vi "Write_Results_file.vi"(0 "Experiment start time":dbl, 1 "Experiment End time":dbl, 3 "Setup filename":string) -> ()   [LabVIEW 2022 SP3]
uses:
  Controls/Post_Process.ctl
  Controls/Inst_type.ctl
  Controls/Global_mode.ctl
  <vilib>/Analysis/baseanly.llb/Mean (DBL).vi
  Globals/Meas_global.vi
  Globals/Trav_pos_global.vi
  Globals/Dynamic_call_global.ph.vi
  <vilib>/Analysis/NI_AALBase.lvlib
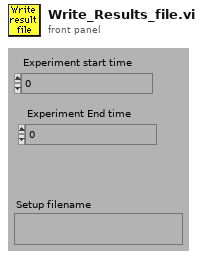
[diagram p1: front panel]
types:
  T1 = typedef "Post_Process.ctl" = enum16{"Take New Data", "Post Process Raw Data File"}
  T2 = enum16{"Save no data", "Save data in new files", "Save data in existing files"}
  T3 = typedef "Inst_type.ctl" = enum16{"Raw voltage", "Raw with zero offsetting", "Propeller anemometer", "Pressure Transducer", "Pitot-static tube", "Hot wire", "Cross wire 1", "Cross wire 2", "Generic Linear", "Generic Polynomial", "Generic BackPoly", "Fast FID", "Thermocouple", "Cold wire", "Pulsed Wire", "LDA Vel", "LDA Tran time", "LDA Arr time", "Microphone"}
  T4 = typedef "Global_mode.ctl" = enum16{"Read Global", "Load Global From File", "Write Global to File"}
  T5 = typedef "Analysis_info_cluster.ctl" = cluster{"Colour":u32, "Inst type":T3, "Inst name":string, "Symbol":string, "Code name":string, "Extra Info":string, "Inst Array":T6, "Extra Titles":string[], "Extra Values":string[], "U":dbl, "u^2":dbl, "u^3":dbl, "u^4":dbl, "Skew_u":dbl, "Kurt_u":dbl, "Sd Error in Mean":dbl, "% u'/U":dbl, "X":dbl, "Y":dbl, "Z":dbl, "Timescale integral Estimate":dbl, "Sd Error in Variance":dbl, "Calib File":path, "Calib Constants":dbl[], "Output Position":bool, "Stats":enum16{"None", "Basic", "Full"}, "Av Sampling Rate":dbl, "Av No of Samples":dbl, "Total Meas Time (s)":dbl, "ADAM Ch Name":string, "Max value":dbl, "Min value":dbl, "Req Sample Rate Hz":dbl, "Sync Delay Time (s)":dbl, "Ch No":i16, "Device":string, "Use Latest Calib":bool, "Port":string, "Metadata Ch Names":string[], "Metadata Ch Values":string[], "Label":string, "chState":T7}
  T6 = typedef "Instrument_Array.ctl" = enum16{"PWA", "LDA", "Analogue"}
  T7 = typedef "channelState.ctl" = enum32{"No Selection", "Solo", "Mute"}
  T8 = typedef "File Update Cluster.ctl" = cluster{"File Path":path, "Rows to Add":i32[], "Extra Ch Names":string[], "Extra Ch Values":string[], "Initial Header String":string, "Separation Character":enum16{"Tab", "Comma"}}
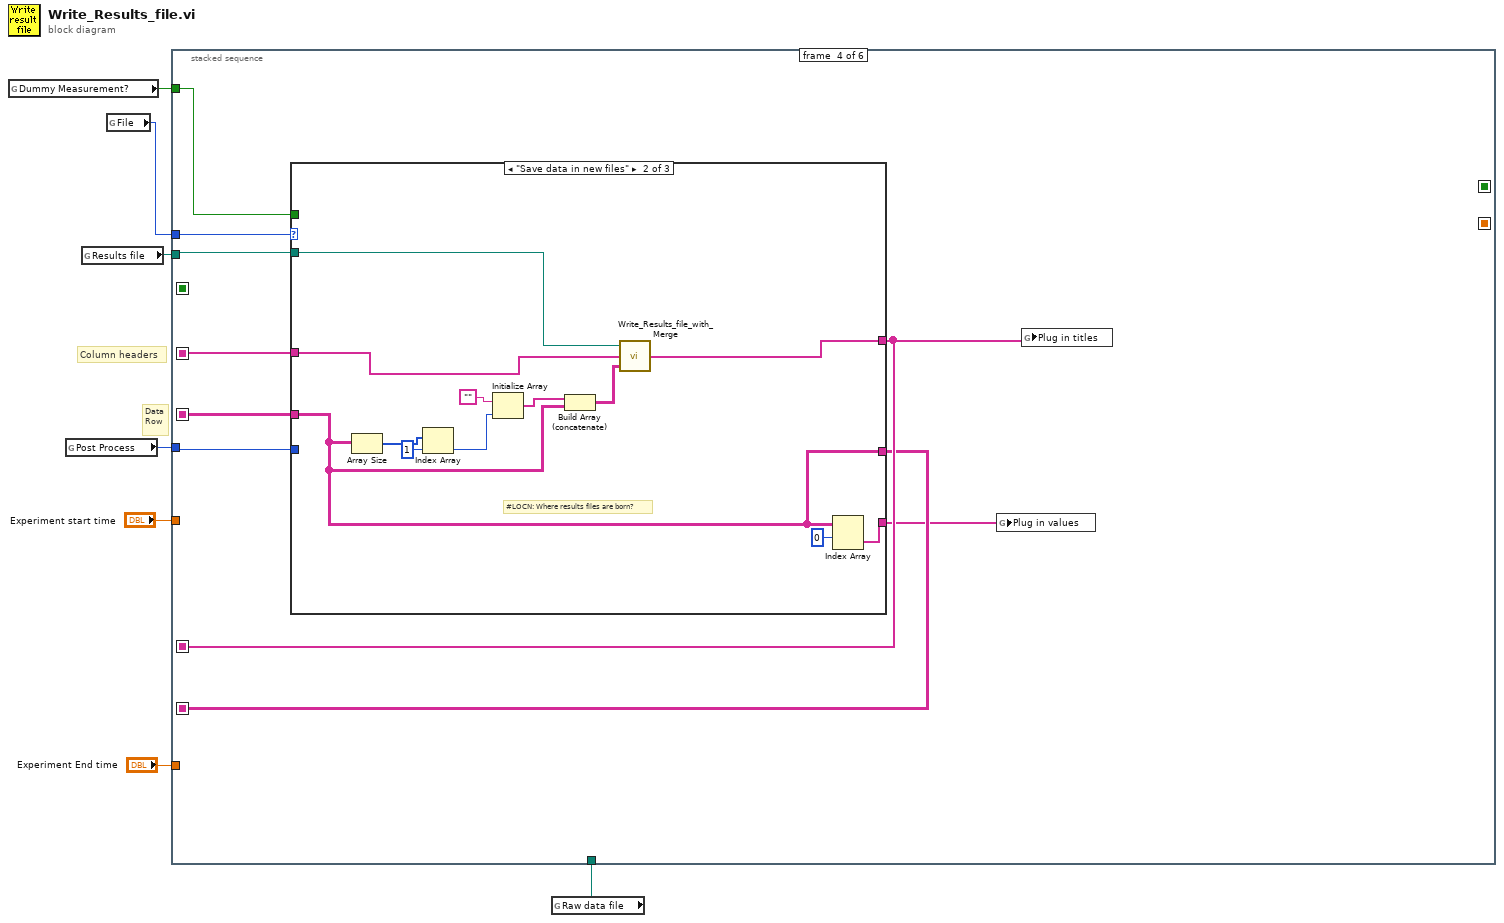
[diagram p0: block diagram]
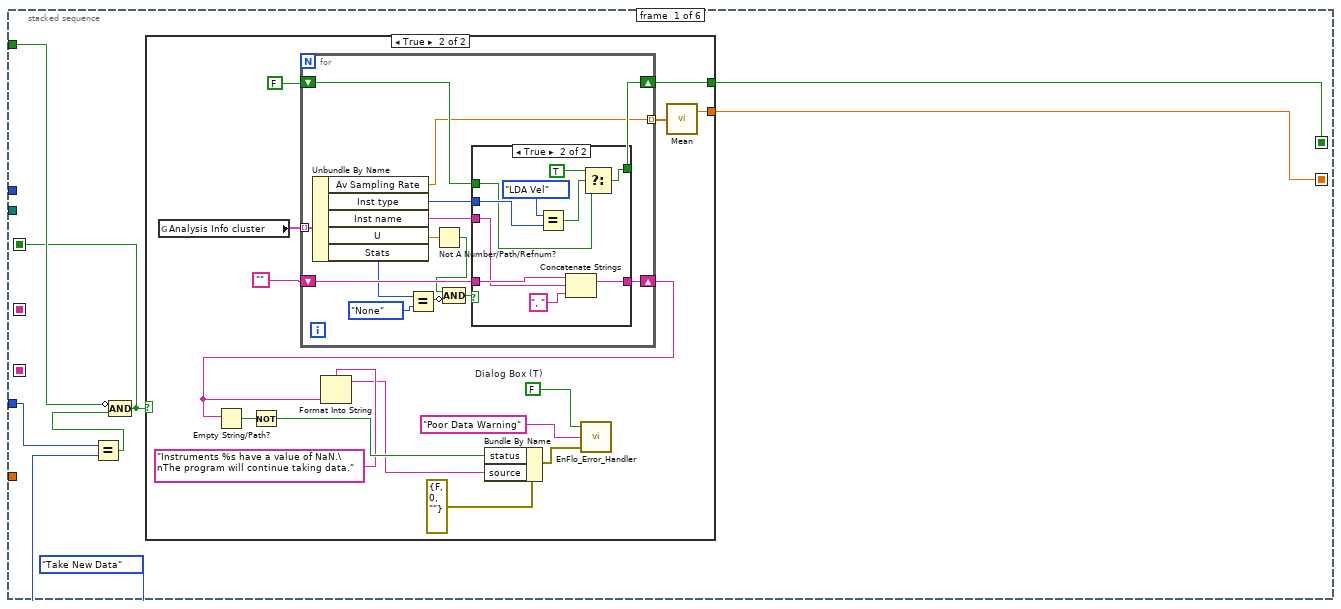
[diagram p2: hidden frame]
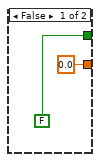
[diagram p3: hidden frame]
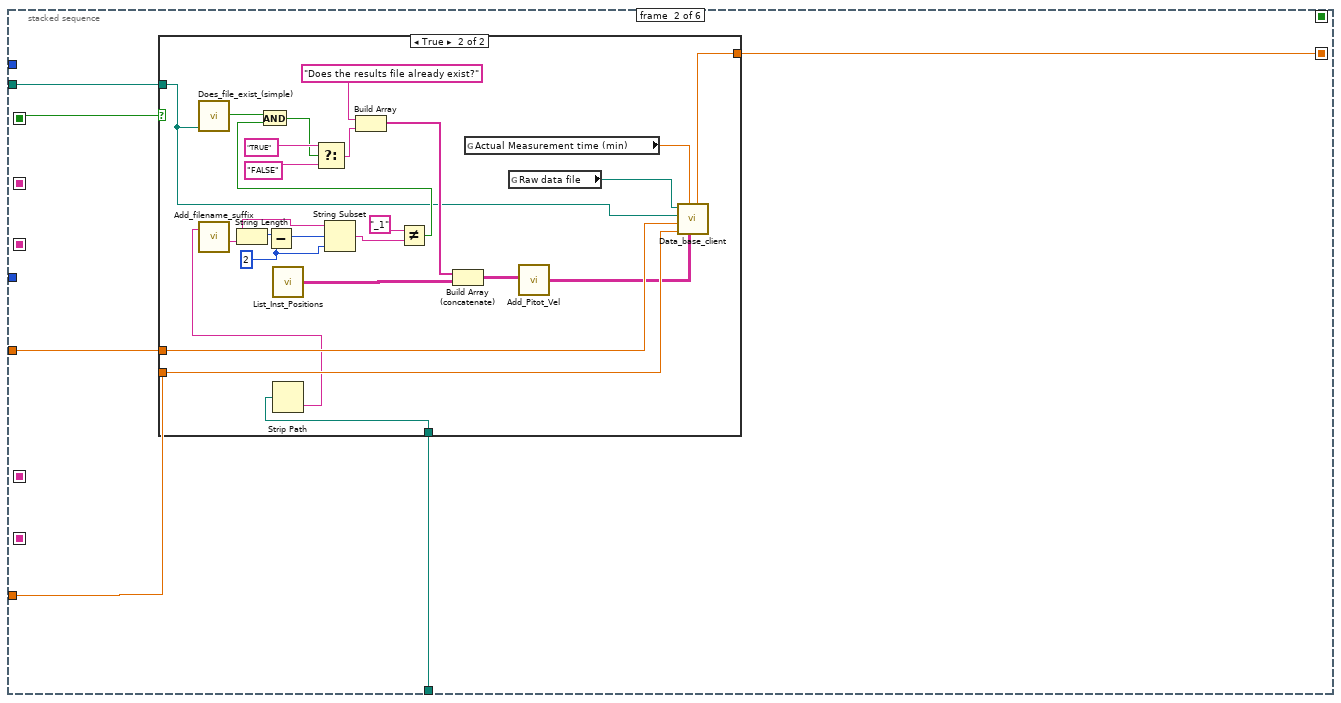
[diagram p5: hidden frame]
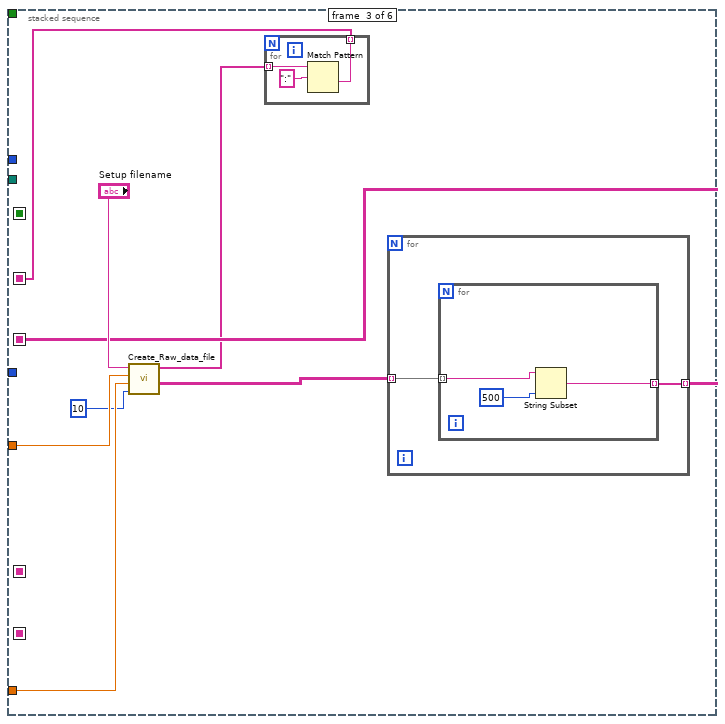
[diagram p7: hidden frame]
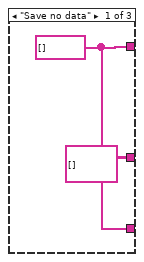
[diagram p8: hidden frame]
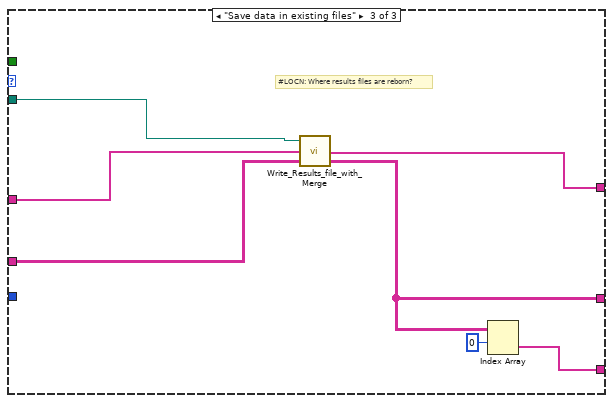
[diagram p9: hidden frame]
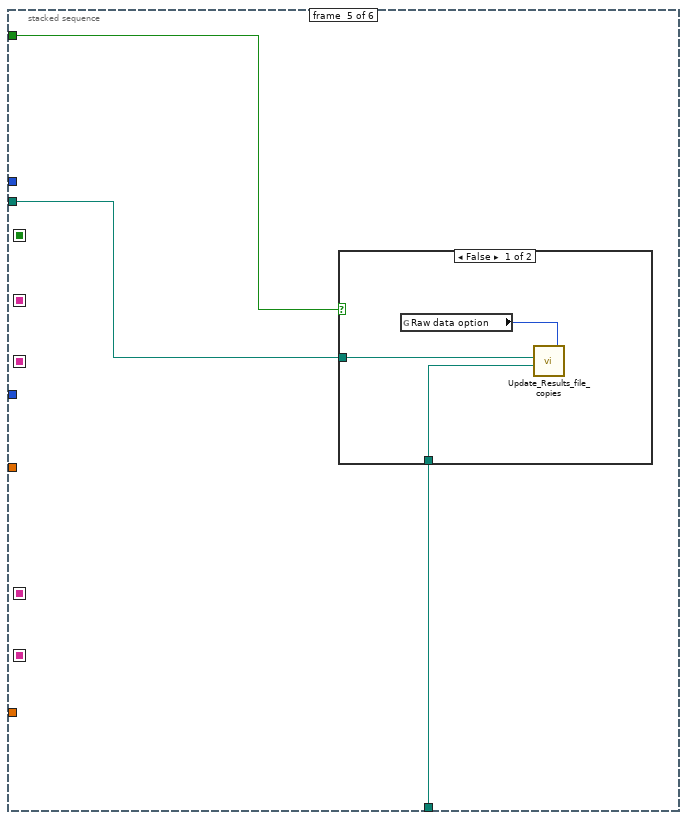
[diagram p10: hidden frame]
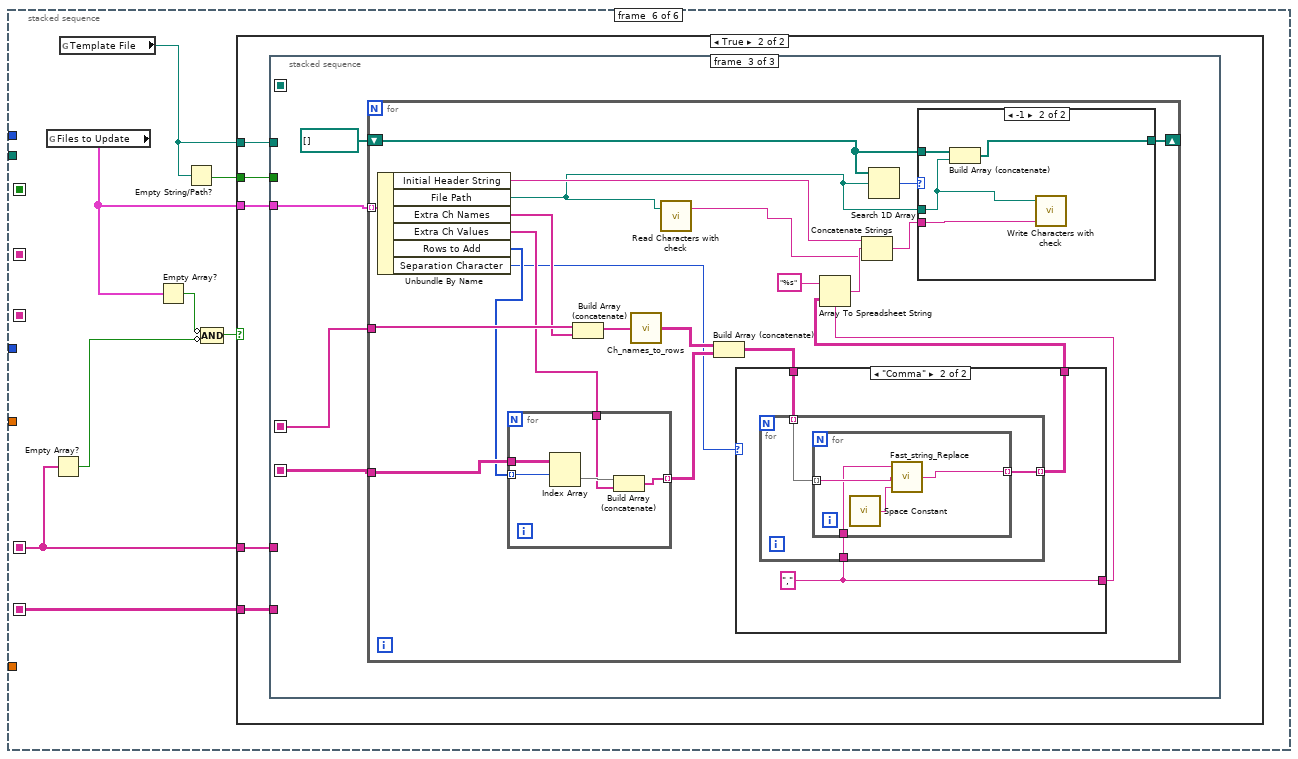
[diagram p12: hidden frame]
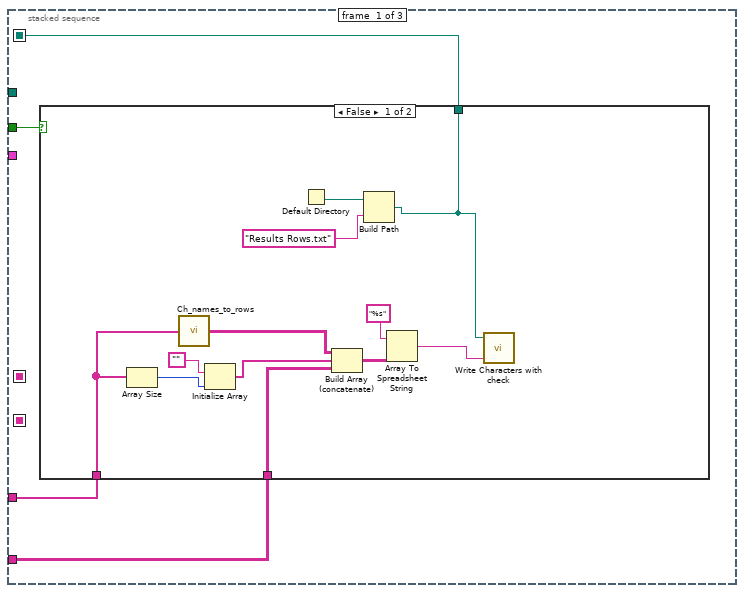
[diagram p14: hidden frame]
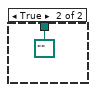
[diagram p15: hidden frame]
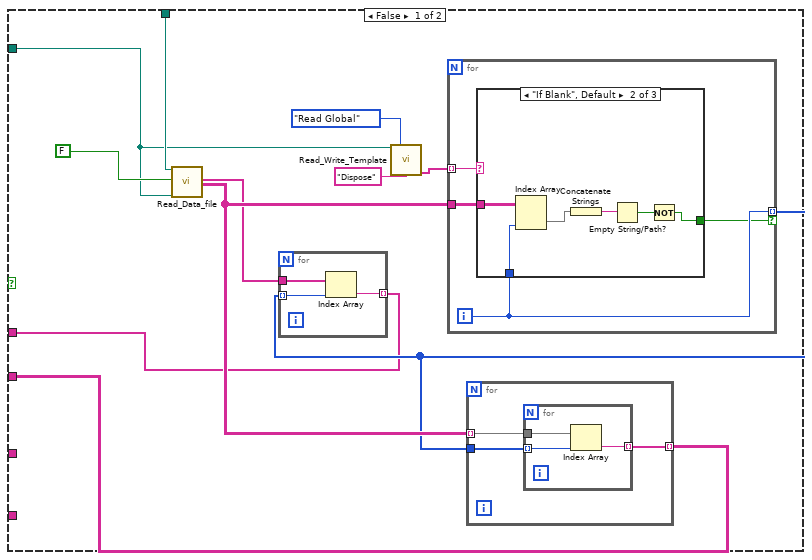
[diagram p17: hidden frame]
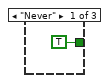
[diagram p18: hidden frame]
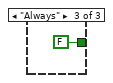
[diagram p19: hidden frame]
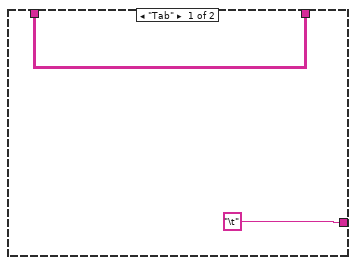
[diagram p20: hidden frame]
diagram:
  # "Data\nRow"
  # "Column headers"
  n1 = global read "Trav_pos_global.vi" "Dummy Measurement?"() -> (w1:bool)
  n2 = global read "Meas_global.vi" "Post Process"() -> (w3:T1)
  n3 = global read "Meas_global.vi" "Results file"() -> (w2:path)
  n4 = global read "Meas_global.vi" "File"() -> (w7:T2)
  n5 = global read "Meas_global.vi" "Raw data file"() -> (w6:path)
  n6 = stacked-sequence {
    seq-local: [_ _ w89 _ _ _] -> [_ _ _ w112 _ _]
    seq-local: [_ _ w91 _ _ _] -> [_ _ _ w111 _ _]
    seq-local: [w10 _ _ _ _ _] -> [_ w60 _ _ _ _]
    seq-local: [w9 _ _ _ _ _] -> [_ _ _ _ _ _]
    seq-local: [w8 _ _ _ _ _] -> [_ w58 _ _ _ _]
    seq-local: [_ _ _ w107 _ _] -> [_ _ _ _ _ w145]
    seq-local: [_ _ _ w106 _ _] -> [_ _ _ _ _ w144]
    tunnel: w7 -> [_ _ _ w113 _ _]
    tunnel: w6 -> [_ w59 _ _ w137 _]
    tunnel: "Experiment start time" -> [_ w63 w96 _ _ _]
    tunnel: "Experiment End time" -> [_ w62 w95 _ _ _]
    tunnel: w3 -> [w13 _ _ w110 _ _]
    tunnel: w2 -> [_ w61 _ w109 w136 _]
    tunnel: w1 -> [w11 _ _ w108 w135 _]
    frame #0 {
      n7 = Equal?(x=w13, y=Post_Process."Take New Data" ("Post Process")) -> (x = y?=w12:bool)
      n8 = Compound Arithmetic op=AND(invert w11, w12) -> (w10:bool)
      n9 = case shown="True" w10 {
        tunnel: [FALSE w19] -> w9
        tunnel: [0.0 ("mean") w17] -> w8
        frame False {
        }
        frame True {
          w28 = FALSE  # Dialog Box (T)
          n10 = global read "Meas_global.vi" "Analysis Info cluster"() -> (w31:T5[])
          n11 = for {
            tunnel: w31 -> [w45] mode=indexing
            shift-right: [w41] -> w23
            shift-left: "" -> [w43]
            shift-right: [w39] -> w19
            shift-left: FALSE -> [w38]
            tunnel: [w37] -> w18 mode=indexing
            n12 = Unbundle By Name(w45) -> ("Av Sampling Rate"=w37:dbl, "Inst type"=w40:T3, "Inst name"=w42:string, "U"=w44:dbl, "Stats"=w35:enum16{"None", "Basic", "Full"})
            n13 = Equal?(x=w35, y=enum16{"None", "Basic", "Full"}."None" ("Stats")) -> (x = y?=w34:bool)
            n14 = Not A Number/Path/Refnum?(number/path/refnum=w44) -> (NaN/Path/Refnum?=w33:bool)
            n15 = Compound Arithmetic op=AND(w33, invert w34) -> (w32:bool)
            n16 = case shown="True" w32 {
              tunnel: w43 -> [w47 w57]
              tunnel: w42 -> [_ w56]
              tunnel: [w47 w54] -> w41
              tunnel: w40 -> [_ w52]
              tunnel: [w46 w49] -> w39
              tunnel: w38 -> [w46 w48]
              frame False {
              }
              frame True {
                n17 = Equal?(x=Inst_type."LDA Vel" ("Inst type"), y=w52) -> (x = y?=w51:bool)
                n18 = Concatenate Strings(w57, w56, ", " ("Substring")) -> (w54:string)
                n19 = Select(t=TRUE, s=w51, f=w48) -> (s? t:f=w49:bool)
              }
            }
          }
          n20 = Empty String/Path?(string/path=w23) -> (empty?=w25:bool)
          n21 = Not(x=w25) -> (.not. x?=w24:bool)
          n22 = Format Into String(format string="Instruments %s have a value of NaN.\nThe program will continue taking data." ("Format String"), w23) -> (resulting string=w21:string)  [unwired: 2 in, 1 out]
          n23 = Bundle By Name(cluster=errorcluster {"status"=FALSE, "code"=0, "source"=""} ("error in (no error)"), "status"=w24, "source"=w21) -> (w26:errorcluster)
          n24 = call "EnFlo_Error_Handler.vi"("error in (no error)"=w26, "Error Type"="Poor Data Warning", "Dialog Box (F)"=w28) -> ()  [unwired: 3 out]
          n25 = call-poly <vilib>:"Mean.vi"("X"=w18) -> ("mean"=w17:dbl)  [unwired: 1 out]
        }
      }
    }
    frame #1 {
      n26 = case shown="True" w60 {
        tunnel: w63 -> [_ w87]
        tunnel: w62 -> [_ w86]
        tunnel: w61 -> [_ w66]
        tunnel: w59 -> [_ w77]
        tunnel: w58 -> [_ w64]
        frame False {
        }
        frame True {
          w72 = 2 ("y")
          n27 = call "Does_file_exist_(simple).vi"("Pathname"=w66) -> ("exists?"=w69:bool)
          n28 = call "List_Inst_Positions.vi"() -> ("Position Info"=w81:string[][])  [unwired: 1 in]
          n29 = Strip Path(path=w77) -> (name=w76:string)  [unwired: 1 out]
          n30 = call "Add_filename_suffix.vi"("Filename"=w76) -> ("Base name"=w75:string)  [unwired: 1 in, 3 out]
          n31 = String Length(string=w75) -> (length=w74:i32)
          n32 = Subtract(x=w74, y=w72) -> (x-y=w73:i32)
          n33 = String Subset(string=w75, offset (0)=w73, length (rest)=w72) -> (substring=w71:string)
          n34 = Not Equal?(x="_1", y=w71) -> (x != y?=w68:bool)
          n35 = And(x=w69, y=w68) -> (x .and. y?=w67:bool)
          n36 = Select(t="TRUE", s=w67, f="FALSE") -> (s? t:f=w84:string)
          n37 = Build Array("Does the results file already exist?", w84) -> (w80:string[])
          n38 = Build Array (concatenate)(w80, w81) -> (w79:string[][])
          n39 = global read "Meas_global.vi" "Actual Measurement time (min)"() -> (w88:dbl)
          n40 = global read "Meas_global.vi" "Raw data file"() -> (w65:path)
          n41 = call "Add_Pitot_Vel.vi"("Channels from Client In"=w79) -> ("Channels from Client Out"=w78:string[][])
          n42 = call "Data_base_client.vi"("Average Sampling freq"=w64, "Channels from Client"=w78, "Average Meas Time (min)"=w88, "End time"=w86, "Start time"=w87, "Results File Pathname"=w66, "Raw Data Pathname"=w65) -> ()  [unwired: 4 out]
        }
      }
    }
    frame #2 {
      n43 = call "Create_Raw_data_file.vi"("Setup filename"="Setup filename", "Start time"=w96, "End time"=w95, "No of averages"=10) -> ("Column headers"=w90:string[], "Values"=w92:string[][])  [unwired: 2 in, 1 out]
      n44 = for {
        tunnel: w90 -> [w99] mode=indexing
        tunnel: [w97] -> w89 mode=indexing
        n45 = Match Pattern(string=w99, regular expression=":") -> (after substring=w97:string)  [unwired: 1 in, 3 out]
      }
      n46 = for {
        tunnel: w92 -> [w101] mode=indexing
        tunnel: [w100] -> w91 mode=indexing
        n47 = for {
          tunnel: w101 -> [w103] mode=indexing
          tunnel: [w102] -> w100 mode=indexing
          n48 = String Subset(string=w103, length (rest)=500 ("y")) -> (substring=w102:string)  [unwired: 1 in]
        }
      }
    }
    frame #3 {
      n49 = case shown="\"Save data in new files\"" w113 {
        tunnel: w112 -> [_ w124 w134]
        tunnel: w111 -> [_ w118 w133]
        tunnel: w109 -> [_ w125 w132]
        tunnel: w110 -> [_ _ _]
        tunnel: [w115 w127 w131] -> w105
        tunnel: [w115 w123 w130] -> w107
        tunnel: w108 -> [_ _ _]
        tunnel: [string[][] [] ("Values Out") w118 w128] -> w106
        frame "Save no data" {
          w115 = string[] [] ("Merged Channels")
        }
        frame "Save data in new files" {
          # "#LOCN: Where results files are born?"
          n50 = Array Size(array=w118) -> (size(s)=w122:i32[])
          n51 = Index Array(array=w122, index=1) -> (element=w120:i32)
          n52 = Initialize Array("", w120) -> (w117:string[])
          n53 = Build Array (concatenate)(w117, w118) -> (w116:string[][])
          n54 = call "Write_Results_file_with_Merge.vi"("Values In"=w116, "Channel Names in"=w124, "Filename"=w125) -> ("Channels Names Out"=w123:string[])  [unwired: 1 in, 1 out]
          n55 = Index Array(array=w118, index (row)=0) -> (element=w127:string[])  [unwired: 1 in]
        }
        frame "Save data in existing files" {
          # "#LOCN: Where results files are reborn?"
          n56 = call "Write_Results_file_with_Merge.vi"("Values In"=w133, "Channel Names in"=w134, "Filename"=w132) -> ("Values Out"=w128:string[][], "Channels Names Out"=w130:string[])  [unwired: 1 in]
          n57 = Index Array(array=w128, index (row)=0) -> (element=w131:string[])  [unwired: 1 in]
        }
      }
      n58 = global write "Dynamic_call_global.ph.vi" "Plug in values"(w105) -> ()
      n59 = global write "Dynamic_call_global.ph.vi" "Plug in titles"(w107) -> ()
    }
    frame #4 {
      n60 = case shown="False" w135 {
        tunnel: w137 -> [w140 _]
        tunnel: w136 -> [w138 _]
        frame False {
          n61 = global read "Meas_global.vi" "Raw data option"() -> (w139:enum16{"Save raw data", "Raw data not saved"})
          n62 = call "Update_Results_file_copies.vi"("Raw data option"=w139, "Raw data file"=w140, "Results file"=w138) -> ()  [unwired: 4 out]
        }
        frame True {
        }
      }
    }
    frame #5 {
      n63 = global read "Meas_global.vi" "Files to Update"() -> (w143:T8[])
      n64 = Empty Array?(array=w145) -> (empty?=w148:bool)
      n65 = global read "Meas_global.vi" "Template File"() -> (w141:path)
      n66 = Empty Array?(array=w143) -> (empty?=w147:bool)
      n67 = Empty String/Path?(string/path=w141) -> (empty?=w142:bool)
      n68 = Compound Arithmetic op=AND(invert w147, invert w148) -> (w146:bool)
      n69 = case shown="True" w146 {
        tunnel: w145 -> [_ w153]
        tunnel: w144 -> [_ w152]
        tunnel: w143 -> [_ w151]
        tunnel: w142 -> [_ w150]
        tunnel: w141 -> [_ w149]
        frame False {
        }
        frame True {
          n70 = stacked-sequence {
            seq-local: [w157 _ _] -> [_ w177 _]
            seq-local: [_ w175 _] -> [_ _ w213]
            seq-local: [_ w176 _] -> [_ _ w214]
            tunnel: w153 -> [w155 w172 _]
            tunnel: w152 -> [w156 w171 _]
            tunnel: w151 -> [_ _ w215]
            tunnel: w150 -> [w154 w173 _]
            tunnel: w149 -> [_ w174 _]
            frame #0 {
              n71 = case shown="False" w154 {
                tunnel: [w159 path "" ("appended path")] -> w157
                tunnel: w156 -> [w164 _]
                tunnel: w155 -> [w163 _]
                frame False {
                  n72 = Array Size(array=w163) -> (size(s)=w162:i32)
                  n73 = call "Ch_names_to_rows.vi"("Channel Names"=w163) -> ("3 Row names"=w169:string[][])
                  n74 = Initialize Array("", w162) -> (w160:string[])
                  n75 = Default Directory() -> (w166:path)
                  n76 = Build Array (concatenate)(w169, w160, w164) -> (w167:string[][])
                  n77 = Build Path(base path=w166, name or relative path="Results Rows.txt") -> (appended path=w159:path)
                  n78 = Array To Spreadsheet String(array=w167, 3:"%s" ("format string")) -> (spreadsheet string=w158:string)  [unwired: 1 out]
                  n79 = call "Write Characters with check.vi"("String to Write"=w158, "file (use dialog)"=w159) -> ()  [unwired: 2 in, 1 out]
                }
                frame True {
                }
              }
            }
            frame #1 {
              n80 = case shown="True" w173 {
                tunnel: w177 -> [w188 _]
                tunnel: [w183 w210] -> w176
                tunnel: [w180 w211] -> w175
                tunnel: w174 -> [w178 _]
                tunnel: w172 -> [_ w211]
                tunnel: w171 -> [_ w210]
                frame False {
                  n81 = call "Read_Data_file.vi"("Results file"=w188, "Delete First Rows?"=FALSE, "Template File"=w178) -> ("Ch names Out"=w181:string[], "Channel Values Out"=w184:string[][])  [unwired: 7 in, 8 out]
                  n82 = call "Read_Write_Template.vi"("Template File"=w178, "Mode"=Global_mode."Read Global", "Data type"="Dispose") -> ("1D Info Out"=w185:string[])  [unwired: 5 in, 7 out]
                  n83 = for {
                    tunnel: w185 -> [w201] mode=indexing
                    tunnel: w184 -> [w200]
                    tunnel: [w199] -> w182 mode=indexing if=w198
                    i -> [w199]
                    n84 = case shown="\"If Blank\", Default" w201 {
                      tunnel: w200 -> [_ w208 _]
                      tunnel: w199 -> [_ w207 _]
                      tunnel: [TRUE w203 FALSE] -> w198
                      frame "Never" {
                      }
                      frame "If Blank", Default {
                        n85 = Index Array(array=w208, index (col)=w207) -> (element=w206:string[])  [unwired: 1 in]
                        n86 = Concatenate Strings(w206) -> (w205:string)
                        n87 = Empty String/Path?(string/path=w205) -> (empty?=w204:bool)
                        n88 = Not(x=w204) -> (.not. x?=w203:bool)
                      }
                      frame "Always" {
                      }
                    }
                  }
                  n89 = for {
                    tunnel: w182 -> [w191] mode=indexing
                    tunnel: w181 -> [w190]
                    tunnel: [w189] -> w180 mode=indexing
                    n90 = Index Array(array=w190, index=w191) -> (element=w189:string)
                  }
                  n91 = for {
                    tunnel: w182 -> [w194]
                    tunnel: w184 -> [w193] mode=indexing
                    tunnel: [w192] -> w183 mode=indexing
                    n92 = for {
                      tunnel: w194 -> [w197] mode=indexing
                      tunnel: w193 -> [w196]
                      tunnel: [w195] -> w192 mode=indexing
                      n93 = Index Array(array=w196, index=w197) -> (element=w195:string)
                    }
                  }
                }
                frame True {
                }
              }
            }
            frame #2 {
              n94 = for {
                tunnel: w215 -> [w237] mode=indexing
                tunnel: w214 -> [w233]
                tunnel: w213 -> [w231]
                shift-right: [w222] -> _
                shift-left: path[] [] -> [w223]
                n95 = Unbundle By Name(w237) -> ("Initial Header String"=w226:string, "File Path"=w217:path, "Extra Ch Names"=w230:string[], "Extra Ch Values"=w227:string[], "Rows to Add"=w228:i32[], "Separation Character"=w221:enum16{"Tab", "Comma"})
                n96 = for {
                  tunnel: w233 -> [w259]
                  tunnel: w228 -> [w258] mode=indexing
                  tunnel: [w257] -> w232 mode=indexing
                  tunnel: w227 -> [w255]
                  n97 = Index Array(array=w259, index (row)=w258) -> (element=w256:string[])  [unwired: 1 in]
                  n98 = Build Array (concatenate)(w256, w255) -> (w257:string[])
                }
                n99 = Build Array (concatenate)(w231, w230) -> (w229:string[])
                n100 = call "Ch_names_to_rows.vi"("Channel Names"=w229) -> ("3 Row names"=w236:string[][])
                n101 = call "Read Characters with check.vi"("file (use dialog)"=w217) -> ("Read String"=w216:string)  [unwired: 1 in, 1 out]
                n102 = Build Array (concatenate)(w236, w232) -> (w220:string[][])
                n103 = case shown="\"Comma\"" w221 {
                  tunnel: ["\t" ("Separation Character 2") w241] -> w218
                  tunnel: w220 -> [w238 w242]
                  tunnel: [w238 w240] -> w219
                  frame "Tab" {
                  }
                  frame "Comma" {
                    w241 = ","
                    n104 = for {
                      tunnel: w242 -> [w245] mode=indexing
                      tunnel: w241 -> [w244]
                      tunnel: [w243] -> w240 mode=indexing
                      n105 = for {
                        tunnel: w245 -> [w248] mode=indexing
                        tunnel: w244 -> [w247]
                        tunnel: [w246] -> w243 mode=indexing
                        n106 = call <vilib>:"Space Constant.vi"() -> ("String"=w249:string)
                        n107 = call "Fast_string_Replace.vi"("Replace match with:"=w249, "Input String"=w248, "matchThis"=w247) -> ("Output String"=w246:string)  [unwired: 1 in, 1 out]
                      }
                    }
                  }
                }
                n108 = Array To Spreadsheet String(delimiter (Tab)=w218, array=w219, 3:"%s" ("format string")) -> (spreadsheet string=w234:string)
                n109 = Concatenate Strings(w226, w234, w216) -> (w224:string)
                n110 = Search 1D Array(1D array=w223, element=w217) -> (index of element=w225:i32)  [unwired: 1 in]
                n111 = case shown="-1" w225 {
                  tunnel: w224 -> [_ w251]
                  tunnel: w223 -> [w250 w254]
                  tunnel: w217 -> [_ w252]
                  tunnel: [w250 w253] -> w222
                  frame Default {
                  }
                  frame -1 {
                    n112 = Build Array (concatenate)(w254, w252) -> (w253:path[])
                    n113 = call "Write Characters with check.vi"("String to Write"=w251, "file (use dialog)"=w252) -> ()  [unwired: 2 in, 1 out]
                  }
                }
              }
            }
          }
        }
      }
    }
  }
